vi "TTA_Read_Test_List.vi"(0 "Working Directory":path, 11 "error in (no error)":errorcluster) -> (4 "RFIC List":T1, 6 "Tx List":T1 caption="RFIC List", 8 "Rx List":T1 caption="RFIC List", 15 "error out":errorcluster)   [LabVIEW 2016]
uses:
  TTA_Controls/TTA_Control_RFIC_List.ctl
  <vilib>/Utility/config.llb/Read Key (String).vi
  <vilib>/Utility/config.llb/NI_LVConfig.lvlib
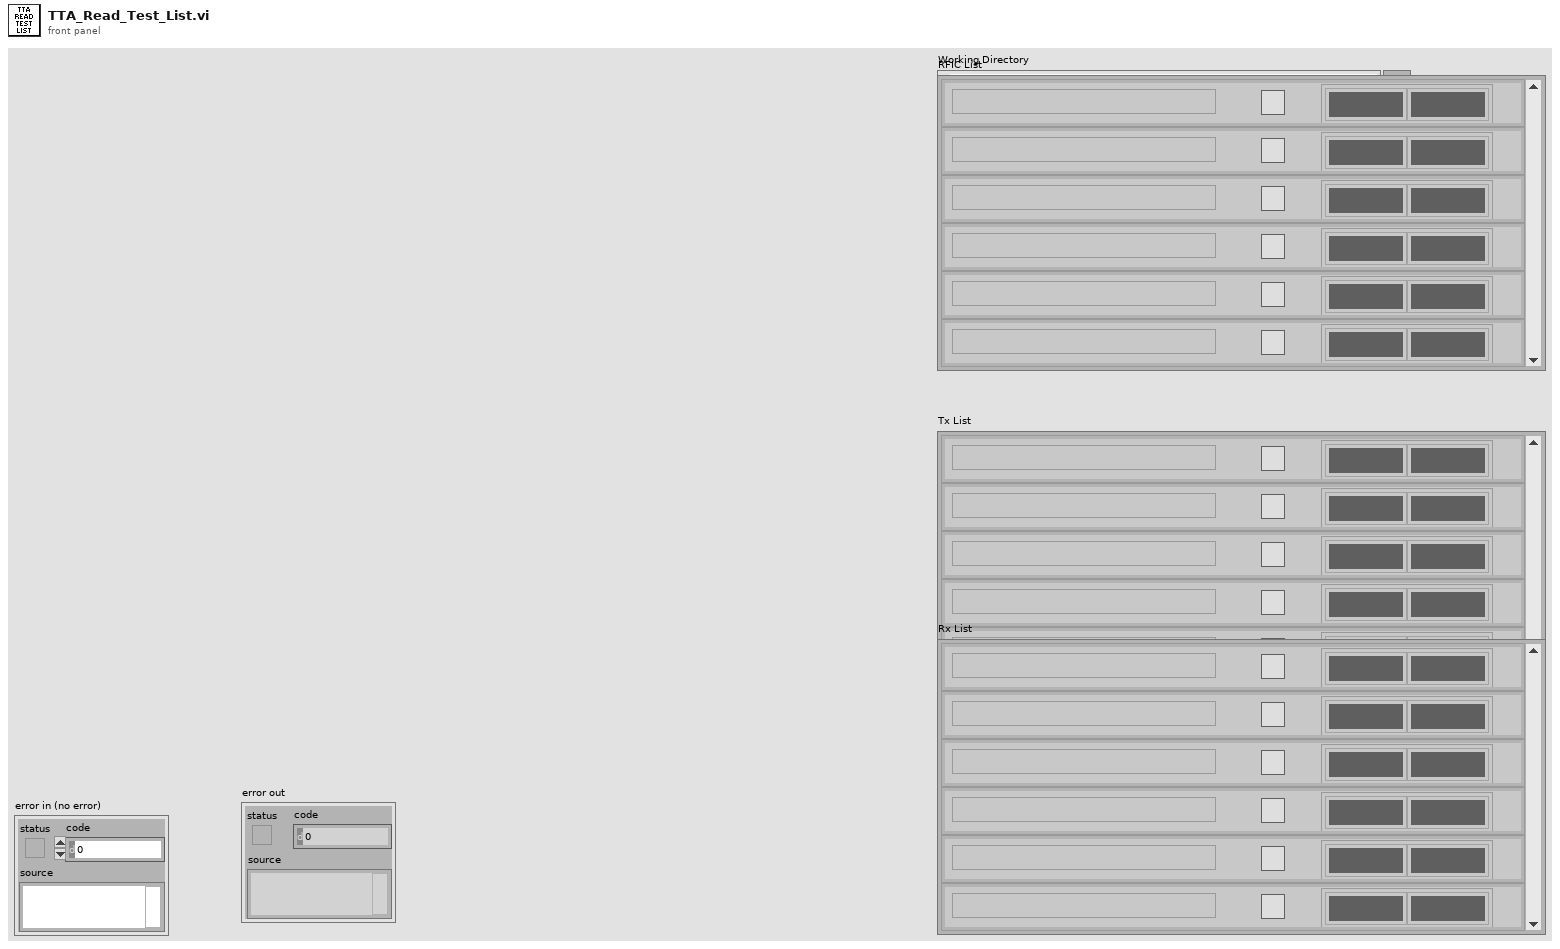
[diagram p1: front panel]
types:
  T1 = typedef "TTA_Control_RFIC_List.ctl" = cluster{"Enable":bool, "Test Description":string, "Status Array":u16[]}[]
  T2 = cluster{"Enable":bool, "Test Description":string, "Status Array":u16[]}
  T3 = typedef "NI_LVConfig.lvlib/Config Data RefNum.ctl" = refnum<k1>
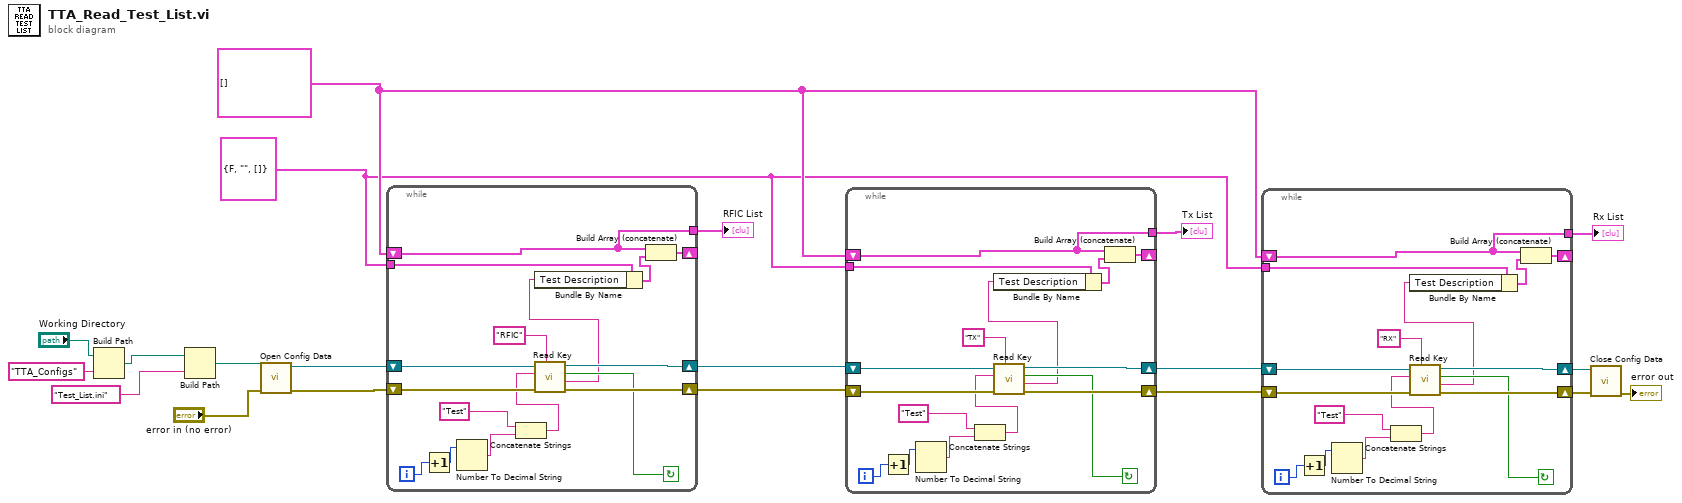
[diagram p0: block diagram]
diagram:
  w1 = T2 {"Enable"=FALSE, "Test Description"="", "Status Array"=[]} ("Cluster")
  w2 = T1 [] ("RFIC List")
  n1 = Build Path(base path="Working Directory", name or relative path="TTA_Configs") -> (appended path=w14:path)
  n2 = Build Path(base path=w14, name or relative path="Test_List.ini") -> (appended path=w12:path)
  n3 = call <vilib>:"Open Config Data.vi"("error in (no error)"="error in (no error)", "configuration file path"=w12) -> ("error out"=w18:errorcluster, "refnum"=w19:T3)  [unwired: 7 in, 1 out]
  n4 = while {
    shift-right: [w34] -> w11
    shift-left: w18 -> [w33]
    shift-right: [w32] -> w10
    shift-left: w19 -> [w36]
    shift-right: [w22] -> _
    shift-left: w2 -> [w21]
    tunnel: w1 -> [w25]
    tunnel: [w21] -> w3
    i -> [w31]
    stop <- w26 continue-if-true
    n5 = Increment(x=w31) -> (x+1=w30:i32)
    n6 = Number To Decimal String(number=w30) -> (decimal integer string=w29:string)  [unwired: 1 in]
    n7 = Concatenate Strings("Test" ("key"), w29) -> (w27:string)
    n8 = call-poly <vilib>:"Read Key.vi"("section"="RFIC", "error in (no error)"=w33, "key"=w27, "refnum"=w36) -> ("error out"=w34:errorcluster, "value"=w24:string, "found?"=w26:bool, "refnum out"=w32:T3)  [unwired: 4 in]
    n9 = Bundle By Name(cluster=w25, "Test Description"=w24) -> (w23:T2)
    n10 = Build Array (concatenate)(w21, w23) -> (w22:T1)
  }
  "RFIC List" <- w3
  n11 = while {
    shift-right: [w50] -> w4
    shift-left: w11 -> [w49]
    shift-right: [w48] -> w5
    shift-left: w10 -> [w52]
    shift-right: [w38] -> _
    shift-left: w2 -> [w37]
    tunnel: w1 -> [w41]
    tunnel: [w37] -> w9
    i -> [w47]
    stop <- w42 continue-if-true
    n12 = Increment(x=w47) -> (x+1=w46:i32)
    n13 = Number To Decimal String(number=w46) -> (decimal integer string=w45:string)  [unwired: 1 in]
    n14 = Concatenate Strings("Test" ("key"), w45) -> (w43:string)
    n15 = call-poly <vilib>:"Read Key.vi"("section"="TX", "error in (no error)"=w49, "key"=w43, "refnum"=w52) -> ("error out"=w50:errorcluster, "value"=w40:string, "found?"=w42:bool, "refnum out"=w48:T3)  [unwired: 4 in]
    n16 = Bundle By Name(cluster=w41, "Test Description"=w40) -> (w39:T2)
    n17 = Build Array (concatenate)(w37, w39) -> (w38:T1)
  }
  "Tx List" <- w9
  n18 = while {
    shift-right: [w66] -> w8
    shift-left: w4 -> [w65]
    shift-right: [w64] -> w7
    shift-left: w5 -> [w68]
    shift-right: [w55] -> _
    shift-left: w2 -> [w54]
    tunnel: w1 -> [w57]
    tunnel: [w54] -> w6
    i -> [w63]
    stop <- w58 continue-if-true
    n19 = Increment(x=w63) -> (x+1=w62:i32)
    n20 = Number To Decimal String(number=w62) -> (decimal integer string=w61:string)  [unwired: 1 in]
    n21 = Concatenate Strings("Test" ("key"), w61) -> (w59:string)
    n22 = call-poly <vilib>:"Read Key.vi"("section"="RX", "error in (no error)"=w65, "key"=w59, "refnum"=w68) -> ("error out"=w66:errorcluster, "value"=w56:string, "found?"=w58:bool, "refnum out"=w64:T3)  [unwired: 4 in]
    n23 = Bundle By Name(cluster=w57, "Test Description"=w56) -> (w53:T2)
    n24 = Build Array (concatenate)(w54, w53) -> (w55:T1)
  }
  "Rx List" <- w6
  n25 = call <vilib>:"Close Config Data.vi"("error in (no error)"=w8, "refnum"=w7) -> ("error out"=→"error out":errorcluster)  [unwired: 8 in, 1 out]
